vi "thcd_get_stat.vi"(8 "err_in":errorcluster, 9 "thcd_b2r":u32, 10 "thcd_delay":u32=500, 11 "thcd_visa":refnum<visa-resource-name>) -> (0 "res 4":T2, 1 "res 3":T2, 2 "res 2":T2, 3 "res_1":T2, 4 "thcd_res_str":string, 5 "thcd_st":bool, 6 "err_out":errorcluster, 7 "thcd_visa":refnum<visa-resource-name>)   [LabVIEW 2013]
uses:
  thcd_controls/ctrl_chn_thcd.ctl
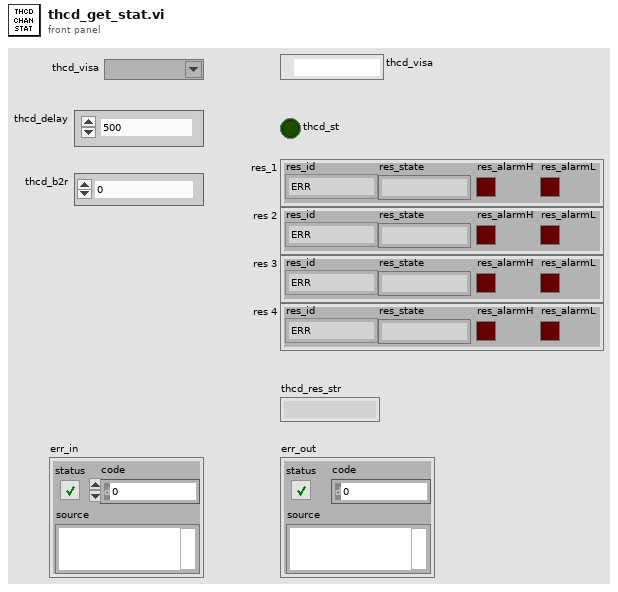
[diagram p1: front panel]
types:
  T1 = typedef "ctrl_chn_thcd.ctl" = enum8{"ERR", "1", "2", "3", "4", "ALL"}
  T2 = cluster{"res_id":T1, "res_alarmH":bool, "res_alarmL":bool, "res_state":string}
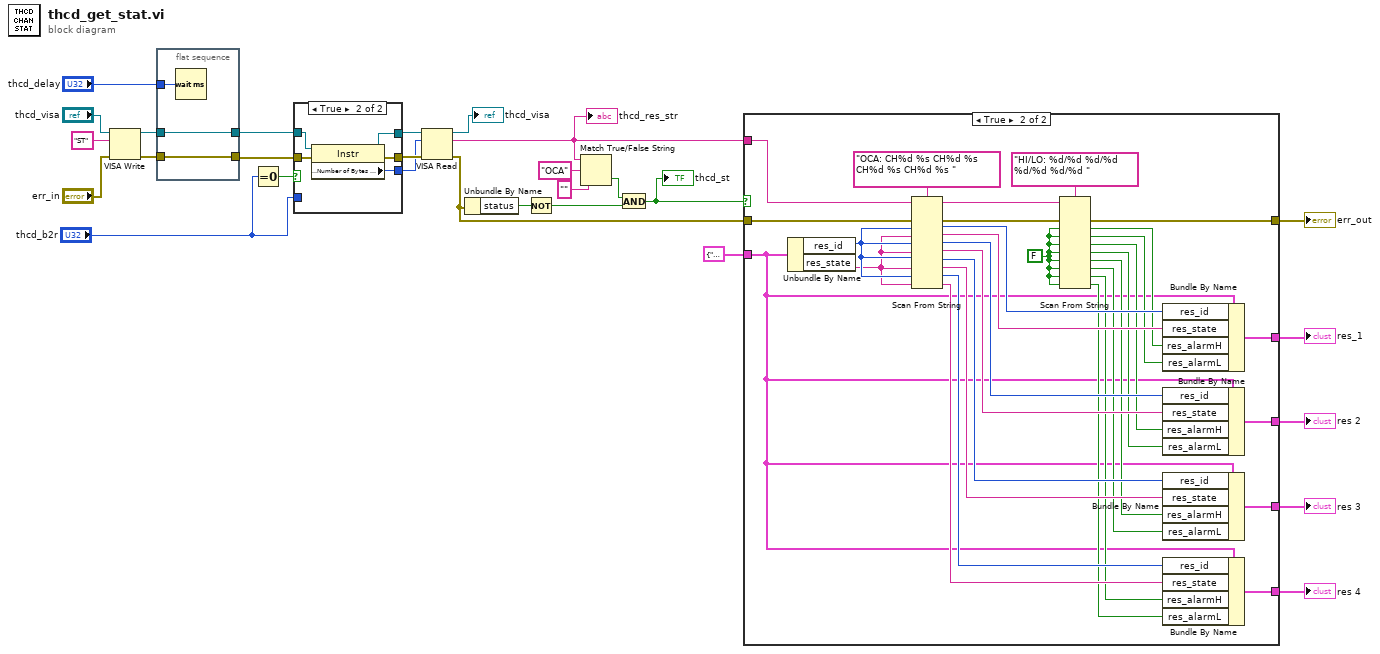
[diagram p0: block diagram]
diagram:
  n1 = VISA Write(VISA resource name="thcd_visa", write buffer="ST" ("format string"), error in (no error)="err_in") -> (VISA resource name out=w27:refnum<visa-resource-name>, error out=w28:errorcluster)  [unwired: 1 out]
  n2 = flat-sequence {
    tunnel: w28 -> [w30]
    tunnel: [w30] -> w15
    tunnel: w27 -> [w29]
    tunnel: [w29] -> w13
    tunnel: "thcd_delay" -> [w31]
    frame #0 {
      n3 = Wait (ms)(milliseconds to wait=w31) -> ()  [unwired: 1 out]
    }
  }
  n4 = Equal To 0?(x="thcd_b2r") -> (x = 0?=w12:bool)
  n5 = case shown="True" w12 {
    tunnel: [w34 w39] -> w10
    tunnel: [w33 w38] -> w14
    tunnel: [w32 w37] -> w9
    tunnel: w15 -> [w33 w36]
    tunnel: w13 -> [w34 w35]
    tunnel: "thcd_b2r" -> [w32 _]
    frame False {
    }
    frame True {
      n6 = property class="Instr"(reference=w35, error in=w36) -> (reference out=w39:refnum<visa-resource-name>, error out=w38:errorcluster, "Serial Settings:Number of Bytes at Serial Port"=w37:u32)
    }
  }
  n7 = VISA Read(VISA resource name=w10, byte count=w9, error in (no error)=w14) -> (VISA resource name out=→"thcd_visa":refnum<visa-resource-name>, read buffer=w22:string, error out=w7:errorcluster)  [unwired: 1 out]
  "thcd_res_str" <- w22
  n8 = Unbundle By Name(w7) -> ("status"=w19:bool)
  n9 = Not(x=w19) -> (.not. x?=w17:bool)
  n10 = Match True/False String(2:"" ("false string"), 3:"OCA" ("true string"), 4:w22) -> (0:w18:bool)  [unwired: 1 out]
  n11 = And(x=w18, y=w17) -> (x .and. y?=w1:bool)
  "thcd_st" <- w1
  n12 = case shown="True" w1 {
    tunnel: [w41 w48] -> w6
    tunnel: T2 {"res_id"=enum."ERR", "res_alarmH"=FALSE, "res_alarmL"=FALSE, "res_state"=""} ("res 2") -> [w41 w44]
    tunnel: [w41 w47] -> w5
    tunnel: [w41 w46] -> w4
    tunnel: [w41 w45] -> w3
    tunnel: w22 -> [_ w69]
    tunnel: w7 -> [w40 w68]
    tunnel: [w40 w42] -> w2
    frame False {
    }
    frame True {
      w49 = FALSE
      n13 = Unbundle By Name(w44) -> ("res_id"=w72:T1, "res_state"=w71:string)
      n14 = Scan From String(format string="OCA: CH%d %s CH%d %s CH%d %s CH%d %s " ("format string 3"), input string=w69, error in=w68, default 1=w72, default 2=w71, default 3=w72, default 4=w71, default 5=w72, default 6=w71, default 7=w72, default 8=w71) -> (remaining string=w67:string, error out=w43:errorcluster, output 1=w65:T1, output 2=w64:string, output 3=w61:T1, output 4=w60:string, output 5=w57:T1, output 6=w56:string, output 7=w53:T1, output 8=w52:string)  [unwired: 1 in, 1 out]
      n15 = Scan From String(format string="HI/LO: %d/%d %d/%d %d/%d %d/%d " ("format string 3"), input string=w67, error in=w43, default 1=w49, default 2=w49, default 3=w49, default 4=w49, default 5=w49, default 6=w49, default 7=w49, default 8=w49) -> (error out=w42:errorcluster, output 1=w63:bool, output 2=w62:bool, output 3=w59:bool, output 4=w58:bool, output 5=w55:bool, output 6=w54:bool, output 7=w51:bool, output 8=w50:bool)  [unwired: 1 in, 2 out]
      n16 = Bundle By Name(cluster=w44, "res_id"=w65, "res_state"=w64, "res_alarmH"=w63, "res_alarmL"=w62) -> (w48:T2)
      n17 = Bundle By Name(cluster=w44, "res_id"=w61, "res_state"=w60, "res_alarmH"=w59, "res_alarmL"=w58) -> (w47:T2)
      n18 = Bundle By Name(cluster=w44, "res_id"=w57, "res_state"=w56, "res_alarmH"=w55, "res_alarmL"=w54) -> (w46:T2)
      n19 = Bundle By Name(cluster=w44, "res_id"=w53, "res_state"=w52, "res_alarmH"=w51, "res_alarmL"=w50) -> (w45:T2)
    }
  }
  "err_out" <- w2
  "res_1" <- w6
  "res 2" <- w5
  "res 3" <- w4
  "res 4" <- w3
